vi "View Song Queue Request.vi"(8 "error in (no error)":errorcluster, 11 "MusicManagerActor in":refnum<class "MusicManagerActor.lvclass">) -> (0 "error out":errorcluster, 3 "MusicManagerActor out":refnum<class "MusicManagerActor.lvclass">)   [LabVIEW 2015, in "MusicManagerActor.lvlib" / "MusicManagerActor.lvclass"]
uses:
  MusicManagerActor.lvclass
  MusicManagerActor.lvclass/MusicManagerActor.ctl
  SongQueueActor/SongQueueActor Messages/Set Visibility Of Queue List Msg/Set Visibility Of Queue List Msg.lvclass
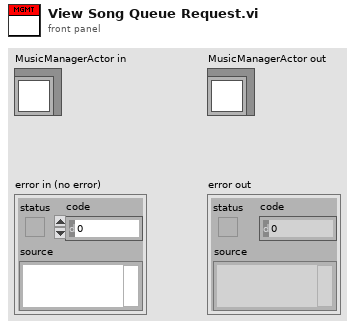
[diagram p1: front panel]
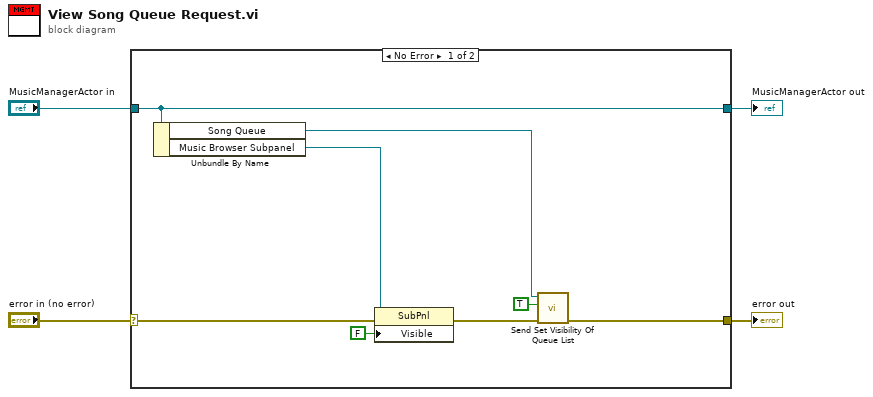
[diagram p0: block diagram]
diagram:
  n1 = case shown="No Error" "error in (no error)" {
    selector: "error in (no error)" -> [w11 w14]
    tunnel: [w6 w14] -> w3
    tunnel: [w12 w13] -> w1
    tunnel: "MusicManagerActor in" -> [w12 w13]
    frame No Error {
      n2 = Unbundle By Name(w12) -> ("Song Queue"=w7:refnum<class "Message Enqueuer.lvclass">, "Music Browser Subpanel"=w10:refnum<vi>)
      n3 = property class="SubPnl"(reference=w10, error in=w11, "Visible"=FALSE) -> (error out=w8:errorcluster)  [unwired: 1 out]
      n4 = call "Send Set Visibility Of Queue List.vi"("error in (no error)"=w8, "Visible"=TRUE, "Message Enqueuer in"=w7) -> ("error out"=w6:errorcluster)  [unwired: 7 in, 1 out]
    }
    frame Error {
    }
  }
  "error out" <- w3
  "MusicManagerActor out" <- w1
